vi "EFW Close.vi"(8 "error in (no error)":errorcluster caption="错误输入（无错误）", 11 "ID":i32) -> (0 "error out":errorcluster caption="错误输出", 3 "function return":u32(ring))   [LabVIEW 2012, in "EFW_filter.lvlib"]
doc: "EFW_API EFW_ERROR_CODE EFWClose(int ID);"
uses:
  <userlib>/EFW_filter/EFW_filter.lvlib
  <userlib>/EFW_filter/EFW_filter.dll
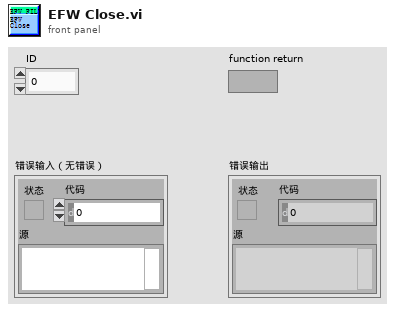
[diagram p1: front panel]
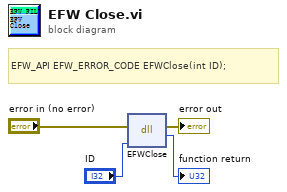
[diagram p0: block diagram]
diagram:
  # "EFW_API\tEFW_ERROR_CODE EFWClose(int ID);"
  n1 = dll-call lib="D:/Program Files (x86)/National Instruments/LabVIEW 2012/user.lib/EFW_filter/EFW_filter.*" fn="EFWClose"(error in="error in (no error)", "ID"="ID") -> (error out=→"error out":errorcluster, →"function return":u32)  [unwired: 3 in, 1 out]
